vi "Error Handler.vi"(8 "error in":errorcluster, 9 "Load Reference?":bool, 11 "Error Queue":refnum<queue>) -> (0 "error out":errorcluster)   [LabVIEW 2020, in "Sensor Interface.lvlib"]
doc: "TEmplate to quickly generate subVIs stubs"
uses:
  Controller/Controls/Module Message.ctl
  Controller/Controls/Application Modules.ctl
  Sensor Interface.lvlib
  Controller/Controller.lvlib
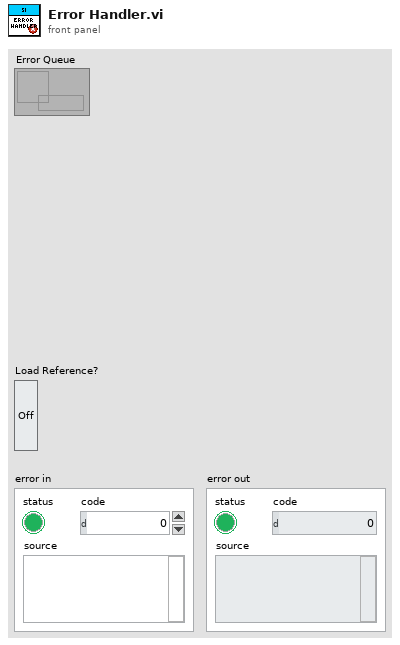
[diagram p1: front panel]
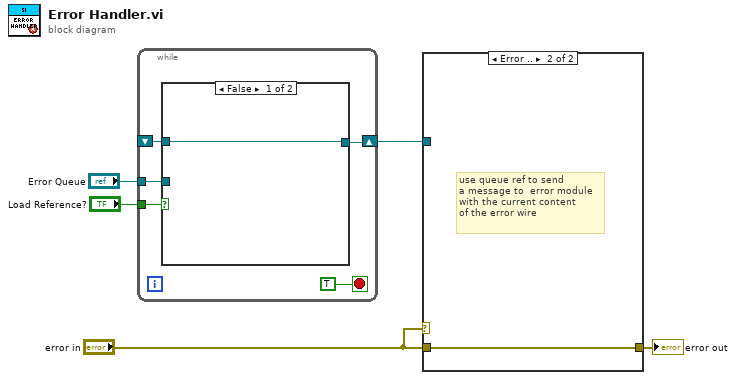
[diagram p0: block diagram]
diagram:
  n1 = while {
    tunnel: "Load Reference?" -> [w9]
    tunnel: "Error Queue" -> [w8]
    shift-right: [w7] -> w1
    shift-left: _ -> [w6]
    stop <- TRUE stop-if-true
    n2 = case shown="False" w9 {
      tunnel: w8 -> [_ w12]
      tunnel: [w11 w12] -> w7
      tunnel: w6 -> [w11 _]
      frame False {
      }
      frame True {
      }
    }
  }
  n3 = case shown="Error .." "error in" {
    tunnel: [w13 w14] -> w5
    tunnel: "error in" -> [w13 w14]
    tunnel: w1 -> [_ _]
    frame No Error {
    }
    frame Error {
      # "use queue ref to send\na message to  error module\nwith the current content \nof the error wire"
    }
  }
  "error out" <- w5
